vi "Sync Mode.vi"() -> ()   [LabVIEW 2012]
doc: "Este VI apresenta uma interface para que o usuário escolha o modo de sincronização das câmeras."
panel:
  in  "OK Button":bool
  in  "Sync Mode:":T1(radio)
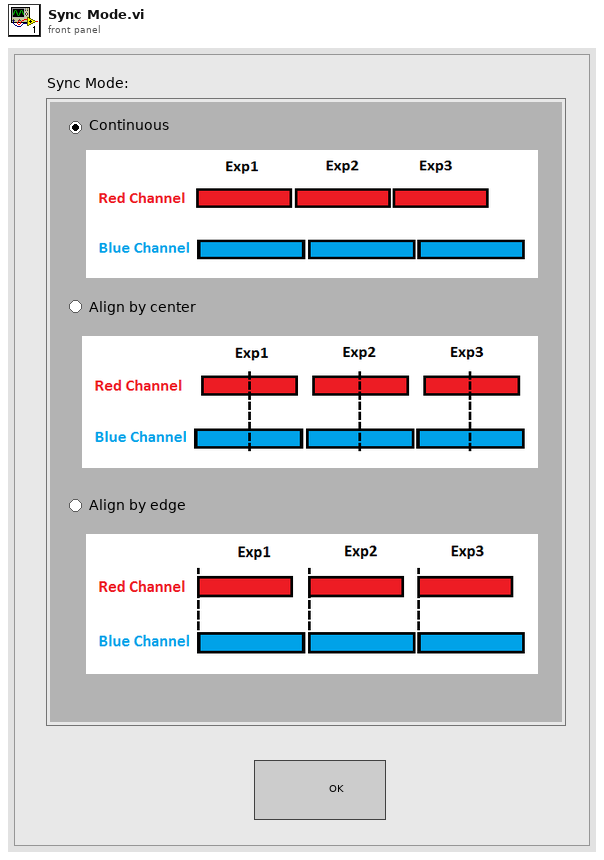
[diagram p1: front panel]
types:
  T1 = enum32{"Radio Selection 1", "Radio Selection 2", "Radio Selection 3"}
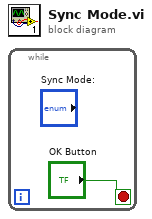
[diagram p0: block diagram]
diagram:
  n1 = while {
    stop <- "OK Button" stop-if-true
  }
